vi "Run.vi"(8 "error in (no error)":errorcluster caption="entrée d'erreur (pas d'erreur)", 11 "Spd_Matrix.lvclass":refnum<class "Spd_Matrix.lvclass">) -> (0 "error out":errorcluster caption="sortie d'erreur", 2 "Data":T1, 3 "Spd_Matrix.lvclass":refnum<class "Spd_Matrix.lvclass">)   [LabVIEW 2020, in "Spd_Matrix.lvclass"]
doc: "Returns :\n\nX : array of shape [n_dim, n_dim]\nThe random symmetric, positive-definite matrix."
uses:
  Spd_Matrix.lvclass
  Spd_Matrix.lvclass/Spd_Matrix.ctl
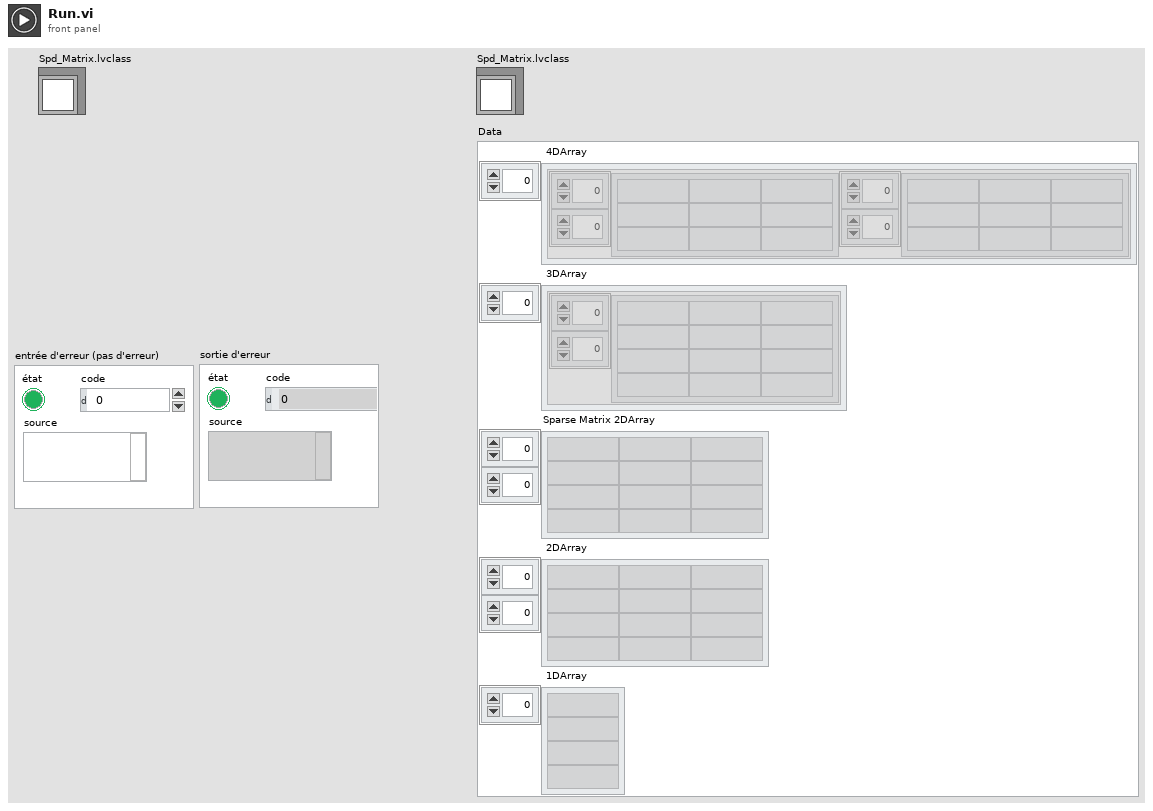
[diagram p1: front panel]
types:
  T1 = cluster{" 4DArray":cluster{"1":string[][], "2":string[][]}[], " 3DArray":cluster{"Tableau":string[][]}[], "Sparse Matrix 2DArray":string[][], " 2DArray":string[][], " 1DArray":string[]}
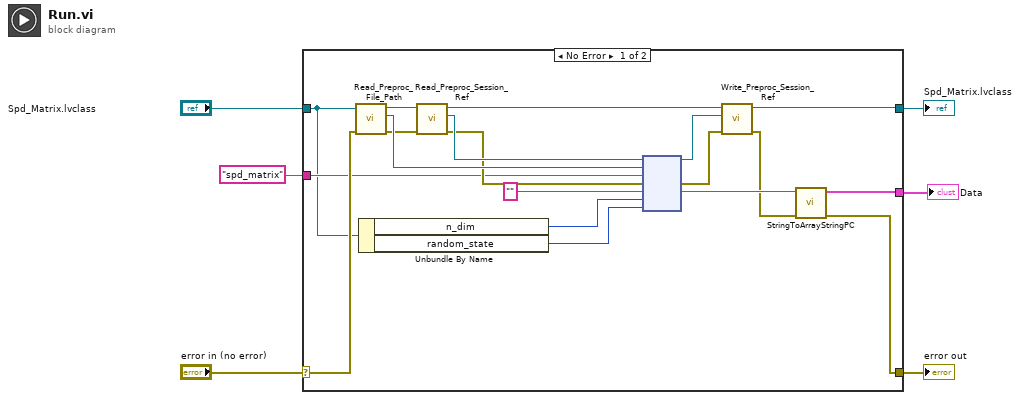
[diagram p0: block diagram]
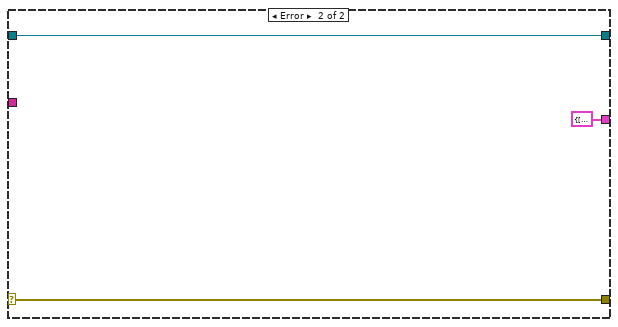
[diagram p2: hidden frame]
diagram:
  n1 = case shown="No Error" "error in (no error)" {
    selector: "error in (no error)" -> [w17 w28]
    tunnel: [w8 w28] -> w5
    tunnel: [w11 w27] -> w3
    tunnel: "Spd_Matrix.lvclass" -> [w15 w27]
    tunnel: "spd_matrix" -> [w16 _]
    tunnel: [w7 T1 {" 4DArray"=[], " 3DArray"=[], "Sparse Matrix 2DArray"=[], " 2DArray"=[], " 1DArray"=[]} ("Data")] -> w1
    frame No Error {
      n2 = call-dynamic "Read_Preproc_File_Path.vi"("error in (no error)"=w17, "Python in"=w15) -> ("error out"=w20:errorcluster, "File_Path"=w23:path, "Python out"=w25:refnum<class "Spd_Matrix.lvclass">)  [unwired: 7 in]
      n3 = Unbundle By Name(w15) -> ("n_dim"=w14:u32, "random_state"=w13:i32)
      n4 = call-dynamic "Read_Preproc_Session_Ref.vi"("error in (no error)"=w20, "Python in"=w25) -> ("error out"=w21:errorcluster, "Session_ref"=w22:refnum<k35>, "Python out"=w24:refnum<class "Spd_Matrix.lvclass">)  [unwired: 7 in]
      n5 = node(w22, w23, w16, w21, "", w14, w13) -> (w18:refnum<k35>, w12:errorcluster, w10:string)  [unwired: 2 in, 2 out]
      n6 = call-dynamic "Write_Preproc_Session_Ref.vi"("error in (no error)"=w12, "Session_ref"=w18, "Python in"=w24) -> ("error out"=w9:errorcluster, "Python out"=w11:refnum<class "Spd_Matrix.lvclass">)  [unwired: 7 in]
      n7 = call "StringToArrayStringPC.vi"("sortie d'erreur"=w9, "Return value"=w10) -> ("sortie d'erreur"=w8:errorcluster, "Data"=w7:T1)  [unwired: 8 in]
    }
    frame Error {
    }
  }
  "error out" <- w5
  "Spd_Matrix.lvclass" <- w3
  "Data" <- w1
